vi "(SubVI)SAI_PANEL_CODIGO.vi"(0 "Modbus Master in":refnum<class "Modbus Master.lvclass">, 3 "SAI":refnum<vi>, 5 "error in (no error)":errorcluster) -> (6 "bypass(F), line (T)":bool, 8 "Tin":u16, 10 "Sin":u16, 12 "Work mode":string, 14 "Modbus Master out":refnum<class "Modbus Master.lvclass">, 15 "Rin":u16, 19 "error out":errorcluster)   [LabVIEW 2024, in "SALICRU_MODBUS.lvlib"]
uses:
  SALICRU_MODBUS.lvlib
  <vilib>/Modbus/master/Modbus Master.lvclass
  <vilib>/Modbus/master/Create Master Instance (TCP).vi
  <vilib>/platform/TimedLoop/XDataNode/XDataNode.xnode
  <vilib>/Platform/TimedLoop/XDataNode/nitl_modes.ctl
  <vilib>/Platform/TimedLoop/XDataNode/XDNodeRunTimeDep.lvlib
  <vilib>/Platform/TimedLoop/XDataNode/wakeup.ctl
  <vilib>/Platform/TimedLoop/XDataNode/timing_clust.ctl
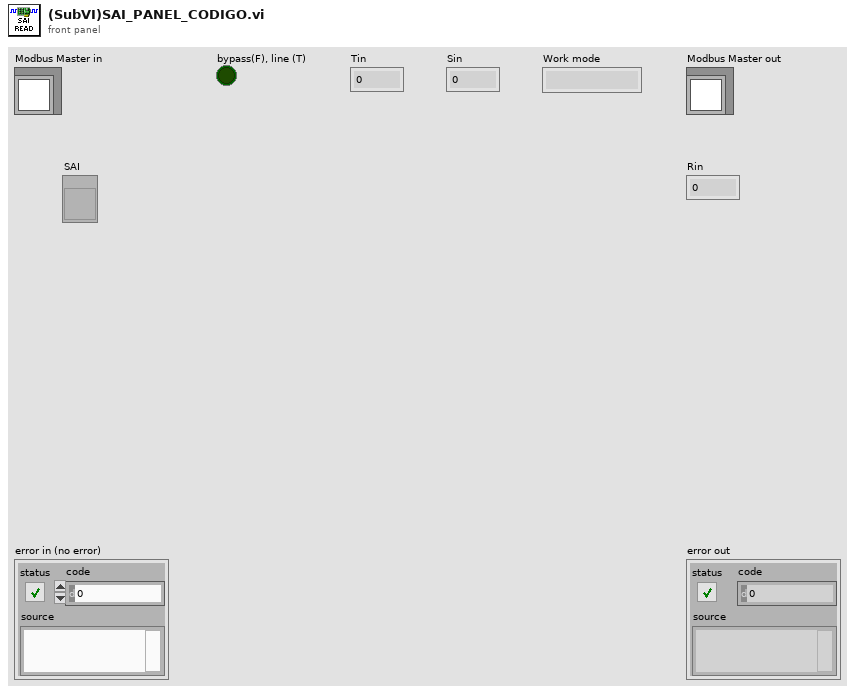
[diagram p1: front panel]
types:
  T1 = typedef "XDNodeRunTimeDep.lvlib/timing_clust.ctl" = cluster{"Expected End [f-1]":u64, "Actual End [f-1]":u64, "Finished Late? [f-1]":bool, "Expected End [i-1]":u64, "Actual End [i-1]":u64, "Finished Late? [i-1]":bool, "Expected Start [i]":u64, "Actual Start [i]":u64, "Expected Start [f]":u64, "Actual Start [f]":u64, "Source Name":string, "Structure Name":string, "Period":i64, "Deadline":i64, "Offset":i64, "Start":i64, "Priority":i32, "Timeout":i32, "Mode":T2, "Wakeup Reason":T3, "Error":errorcluster, "Source Type":string, "Secondary Source Type":string, "Global End Time":u64, "Global Start Time":u64, "Frame Duration":u64, "Iteration Duration":u64, "Assigned CPU":i32, "I/O Scan Engine Mode":u32}
  T2 = typedef "XDNodeRunTimeDep.lvlib/nitl_modes.ctl" = enum32{"No Change", "Process missed periods, maintain original phase", "Discard missed periods, maintain original phase", "Process missed periods, ignore original phase", "Discard missed periods, ignore original phase"}
  T3 = typedef "XDNodeRunTimeDep.lvlib/wakeup.ctl" = enum32{"Normal", "Aborted", "Asynchronous wakeup", "Timing source error", "Timed loop error", "Timeout"}
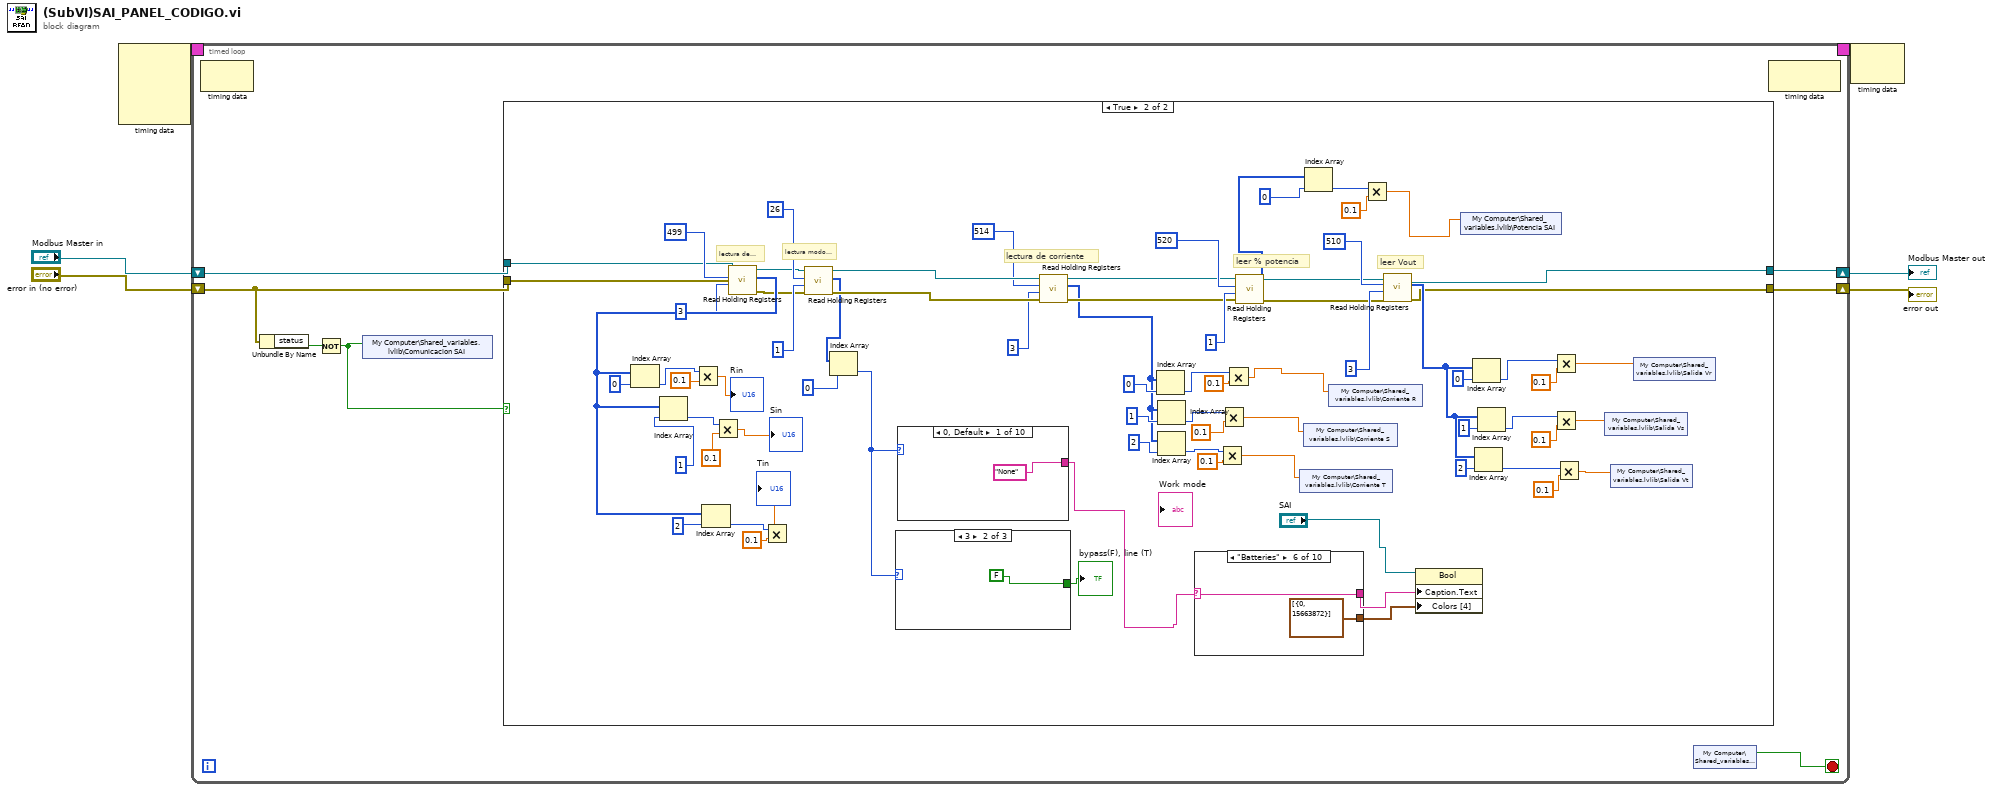
[diagram p0: block diagram]
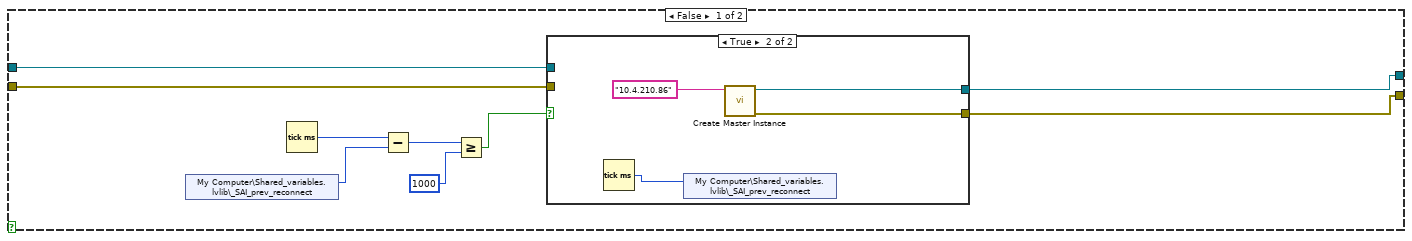
[diagram p2: hidden frame]
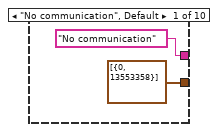
[diagram p4: hidden frame]
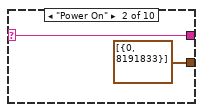
[diagram p5: hidden frame]
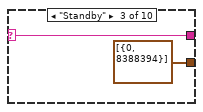
[diagram p6: hidden frame]
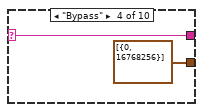
[diagram p7: hidden frame]
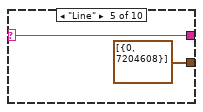
[diagram p8: hidden frame]
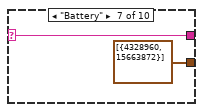
[diagram p9: hidden frame]
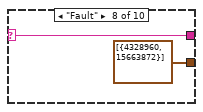
[diagram p10: hidden frame]
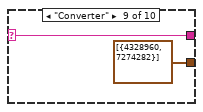
[diagram p11: hidden frame]
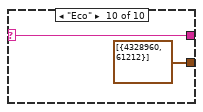
[diagram p12: hidden frame]
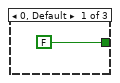
[diagram p13: hidden frame]
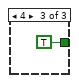
[diagram p14: hidden frame]
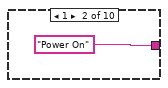
[diagram p15: hidden frame]
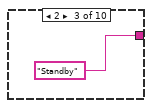
[diagram p16: hidden frame]
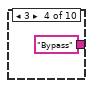
[diagram p17: hidden frame]
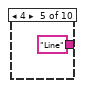
[diagram p18: hidden frame]
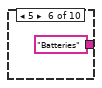
[diagram p19: hidden frame]
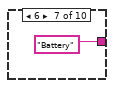
[diagram p20: hidden frame]
diagram:
  n1 = node-c288() -> (w2:T1)  [unwired: 4 in]
  n2 = timed-loop {
    timing: w2 -> [_]
    timing-out: [_] -> w1
    shift-right: [w13] -> w6
    shift-left: "Modbus Master in" -> [w12]
    shift-right: [w10] -> w4
    shift-left: "error in (no error)" -> [w9]
    stop <- w7 stop-if-true
    n3 = node-c288() -> ()  [unwired: 1 in, 1 out]
    n4 = Unbundle By Name(w9) -> ("status"=w11:bool)
    n5 = Not(x=w11) -> (.not. x?=w8:bool)
    n6 = shared-variable "My Computer\\Shared_variables.lvlib\\Comunicacion SAI"(w8) -> ()  [unwired: 1 in, 1 out]
    n7 = case shown="True" w8 {
      tunnel: [w17 w88] -> w13
      tunnel: w12 -> [w15 w42]
      tunnel: [w16 w40] -> w10
      tunnel: w9 -> [w14 w29]
      frame False {
        n8 = shared-variable "My Computer\\Shared_variables.lvlib\\_SAI_prev_reconnect"() -> (w18:u32)  [unwired: 1 in, 1 out]
        n9 = Tick Count (ms)() -> (millisecond timer value=w22:u32)
        n10 = Subtract(x=w22, y=w18) -> (x-y=w21:u32)
        n11 = Greater Or Equal?(x=w21, y=u32 1000) -> (x >= y?=w19:bool)
        n12 = case shown="True" w19 {
          tunnel: [w24 w26] -> w17
          tunnel: [w23 w25] -> w16
          tunnel: w15 -> [w24 _]
          tunnel: w14 -> [w23 _]
          frame False {
          }
          frame True {
            n13 = Tick Count (ms)() -> (millisecond timer value=w28:u32)
            n14 = shared-variable "My Computer\\Shared_variables.lvlib\\_SAI_prev_reconnect"(w28) -> ()  [unwired: 1 in, 1 out]
            n15 = call-poly <vilib>:"Create Master Instance.vi"("address"="10.4.210.86") -> ("error out"=w25:errorcluster, "TCP master instance"=w26:refnum<class "Modbus Master.lvclass">)  [unwired: 9 in]
          }
        }
      }
      frame True {
        # "leer Vout"
        # "leer % potencia"
        # "lectura de corriente"
        # "lectura modos de trabajo"
        # "lectura de tensiones de entrada"
        n16 = call-dynamic "Read Holding Registers.vi"("error in (no error)"=w29, "number of holding registers"=u16 3, "starting address"=u16 499, "Modbus master in"=w42) -> ("error out"=w46:errorcluster, "register values"=w54:u16[], "Modbus master out"=w45:refnum<class "Modbus Master.lvclass">)  [unwired: 5 in]
        n17 = Index Array(array=w54, index=0) -> (element=w61:u16)
        n18 = Index Array(array=w54, index=1) -> (element=w63:u16)
        n19 = Multiply(x=w61, y=0.1) -> (x*y=→"Rin":dbl)
        n20 = Index Array(array=w54, index=2) -> (element=w67:u16)
        n21 = Multiply(x=w63, y=0.1) -> (x*y=→"Sin":dbl)
        n22 = Multiply(x=w67, y=0.1) -> (x*y=→"Tin":dbl)
        n23 = call-dynamic "Read Holding Registers.vi"("error in (no error)"=w46, "number of holding registers"=u16 1, "starting address"=u16 26, "Modbus master in"=w45) -> ("error out"=w92:errorcluster, "register values"=w48:u16[], "Modbus master out"=w91:refnum<class "Modbus Master.lvclass">)  [unwired: 5 in]
        n24 = Index Array(array=w48, index=0) -> (element=w50:u16)
        n25 = case shown="3" w50 {
          tunnel: [FALSE FALSE TRUE] -> w51
          frame 0, Default {
          }
          frame 3 {
          }
          frame 4 {
          }
        }
        "bypass(F), line (T)" <- w51
        n26 = case shown="0, Default" w50 {
          tunnel: ["None" "Power On" "Standby" "Bypass" "Line" "Batteries" "Battery" "Fault" "Converter" "ECO"] -> w31
          frame 0, Default {
          }
          frame 1 {
          }
          frame 2 {
          }
          frame 3 {
          }
          frame 4 {
          }
          frame 5 {
          }
          frame 6 {
          }
          frame 7 {
          }
          frame 8 {
          }
          frame 9 {
          }
        }
        n27 = call-dynamic "Read Holding Registers.vi"("error in (no error)"=w92, "number of holding registers"=u16 3, "starting address"=u16 514, "Modbus master in"=w91) -> ("error out"=w79:errorcluster, "register values"=w58:u16[], "Modbus master out"=w78:refnum<class "Modbus Master.lvclass">)  [unwired: 5 in]
        n28 = Index Array(array=w58, index=0) -> (element=w70:u16)
        n29 = Index Array(array=w58, index=1) -> (element=w72:u16)
        n30 = Index Array(array=w58, index=2) -> (element=w74:u16)
        n31 = case shown="\"Batteries\"" w31 {
          selector: w31 -> [_ w106 w108 w110 w112 w114 w116 w118 w120 w122]
          tunnel: ["No communication" w106 w108 w110 w112 w114 w116 w118 w120 w122] -> w32
          tunnel: [cluster{u32, u32}[] [{0, 13553358}] ("Colors [4]") cluster{u32, u32}[] [{0, 8191833}] ("Colors [4]") cluster{u32, u32}[] [{0, 8388394}] ("Colors [4]") cluster{u32, u32}[] [{0, 16768256}] ("Colors [4]") cluster{u32, u32}[] [{0, 7204608}] ("Colors [4]") cluster{u32, u32}[] [{0, 15663872}] ("Colors [4]") cluster{u32, u32}[] [{4328960, 15663872}] ("Colors [4]") cluster{u32, u32}[] [{4328960, 15663872}] ("Colors [4]") cluster{u32, u32}[] [{4328960, 7274282}] ("Colors [4]") cluster{u32, u32}[] [{4328960, 61212}] ("Colors [4]")] -> w33
          frame "No communication", Default {
          }
          frame "Power On" {
          }
          frame "Standby" {
          }
          frame "Bypass" {
          }
          frame "Line" {
          }
          frame "Batteries" {
          }
          frame "Battery" {
          }
          frame "Fault" {
          }
          frame "Converter" {
          }
          frame "Eco" {
          }
        }
        n32 = Multiply(x=w74, y=0.1) -> (x*y=w37:dbl)
        n33 = Multiply(x=w72, y=0.1) -> (x*y=w38:dbl)
        n34 = Multiply(x=w70, y=0.1) -> (x*y=w39:dbl)
        n35 = call-dynamic "Read Holding Registers.vi"("error in (no error)"=w79, "number of holding registers"=u16 1, "starting address"=u16 520, "Modbus master in"=w78) -> ("error out"=w87:errorcluster, "register values"=w82:u16[], "Modbus master out"=w86:refnum<class "Modbus Master.lvclass">)  [unwired: 5 in]
        n36 = shared-variable "My Computer\\Shared_variables.lvlib\\Corriente T"(w37) -> ()  [unwired: 1 in, 1 out]
        n37 = shared-variable "My Computer\\Shared_variables.lvlib\\Corriente S"(w38) -> ()  [unwired: 1 in, 1 out]
        n38 = Index Array(array=w82, index=0) -> (element=w85:u16)
        n39 = shared-variable "My Computer\\Shared_variables.lvlib\\Corriente R"(w39) -> ()  [unwired: 1 in, 1 out]
        n40 = Multiply(x=w85, y=0.1) -> (x*y=w41:dbl)
        n41 = call-dynamic "Read Holding Registers.vi"("error in (no error)"=w87, "number of holding registers"=u16 3, "starting address"=u16 510, "Modbus master in"=w86) -> ("error out"=w40:errorcluster, "register values"=w93:u16[], "Modbus master out"=w88:refnum<class "Modbus Master.lvclass">)  [unwired: 5 in]
        n42 = property class="Bool"(reference="SAI", "Caption.Text"=w32, "Colors [4]"=w33) -> ()  [unwired: 1 in, 2 out]
        n43 = shared-variable "My Computer\\Shared_variables.lvlib\\Potencia SAI"(w41) -> ()  [unwired: 1 in, 1 out]
        n44 = Index Array(array=w93, index=0) -> (element=w100:u16)
        n45 = Index Array(array=w93, index=2) -> (element=w102:u16)
        n46 = Index Array(array=w93, index=1) -> (element=w101:u16)
        n47 = Multiply(x=w100, y=0.1) -> (x*y=w36:dbl)
        n48 = Multiply(x=w101, y=0.1) -> (x*y=w35:dbl)
        n49 = Multiply(x=w102, y=0.1) -> (x*y=w34:dbl)
        n50 = shared-variable "My Computer\\Shared_variables.lvlib\\Salida Vs"(w35) -> ()  [unwired: 1 in, 1 out]
        n51 = shared-variable "My Computer\\Shared_variables.lvlib\\Salida Vt"(w34) -> ()  [unwired: 1 in, 1 out]
        n52 = shared-variable "My Computer\\Shared_variables.lvlib\\Salida Vr"(w36) -> ()  [unwired: 1 in, 1 out]
      }
    }
    n53 = shared-variable "My Computer\\Shared_variables.lvlib\\Stop"() -> (w7:bool)  [unwired: 1 in, 1 out]
    n54 = node-c288() -> ()  [unwired: 1 in, 1 out]
  }
  "Modbus Master out" <- w6
  "error out" <- w4
  n55 = node-c288(w1) -> ()  [unwired: 1 out]
